vi "Wolna_licz_czas.vi"(8 "error in (no error)":errorcluster, 11 "Array":bool[](array[boolean])) -> (0 "error out":errorcluster, 3 "l.probek":dbl)   [LabVIEW 2013]
doc: "Liczy czastrwania stanu wysokiego\nprzebiegu wzmocnionego"
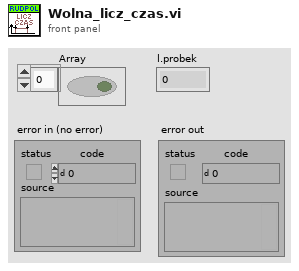
[diagram p1: front panel]
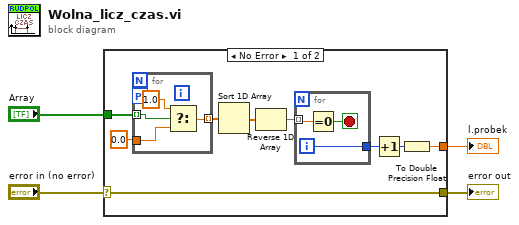
[diagram p0: block diagram]
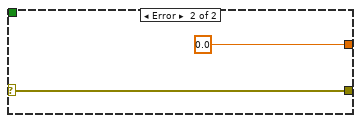
[diagram p2: hidden frame]
diagram:
  n1 = case shown="No Error" "error in (no error)" {
    selector: "error in (no error)" -> [w5 w22]
    tunnel: [w5 w22] -> w4
    tunnel: "Array" -> [w7 _]
    tunnel: [w6 0.0] -> w1
    frame No Error {
      n2 = for {
        tunnel: w7 -> [w20] mode=indexing
        tunnel: 0.0 ("y") -> [w19]
        tunnel: [w17] -> w10 mode=indexing
        workers-P: _ -> [_]
        n3 = Select(t=1.0, s=w20, f=w19) -> (s? t:f=w17:dbl)
      }
      n4 = Sort 1D Array(array=w10) -> (sorted array=w11:dbl[])
      n5 = Reverse 1D Array(array=w11) -> (reversed array=w9:dbl[])
      n6 = for {
        tunnel: w9 -> [w16] mode=indexing
        tunnel: [w14] -> w8
        i -> [w14]
        stop <- w15 stop-if-true
        n7 = Equal To 0?(x=w16) -> (x = 0?=w15:bool)
      }
      n8 = Increment(x=w8) -> (x+1=w13:i32)
      n9 = To Double Precision Float(number=w13) -> (double precision float=w6:dbl)
    }
    frame Error {
    }
  }
  "l.probek" <- w1
  "error out" <- w4
